vi "Set Service map mutex.vi"(10 "semaphore":T1, 11 "CANopen in":refnum<class "CANopen.lvclass">) -> (3 "CANopen out":refnum<class "CANopen.lvclass">)   [LabVIEW 2024]
uses:
  CANopen.lvclass/CANopen.ctl
  CANopen.lvclass
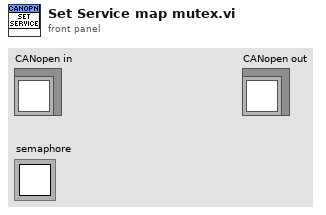
[diagram p1: front panel]
types:
  T1 = typedef "Semaphore RefNum" = refnum<k1>
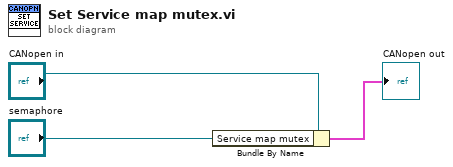
[diagram p0: block diagram]
diagram:
  n1 = Bundle By Name(cluster="CANopen in", "Service map mutex"="semaphore") -> (→"CANopen out":cluster{})
